vi "BonOMM-SAOMM.vi"() -> ()   [LabVIEW 2019] (continued)
                    n5983 = call "format_arcmin2arcsecstr.vi"("RA arcmin"=w2817, "DEC Arcmin"=w2816) -> ("Formatted RA"=w2820:string, "Formatted Dist"=w2818:string, "Formatted DEC"=w2819:string)  [unwired: 11 in]
                    n5984 = Array Max & Min(array=w2824) -> (max value=w2825:sgl)  [unwired: 3 out]
                    n5985 = call "Draw_crosshair.vi"("Image IN"=w2824, "White Value"=w2825) -> ("Image OUT"=w2823:sgl[][])  [unwired: 13 in]
                    n5986 = local write "SubIMG4DSS?"(TRUE ("SubIMG4DSS?")) -> ()
                    n5987 = local write "Cen-Cib-TOT"(w2818) -> ()
                    n5988 = local write "Cen-Cib-RA"(w2820) -> ()
                    n5989 = local write "Cen-Cib-DEC"(w2819) -> ()
                    n5990 = local write "ImageUsage"(w2808) -> ()
                    n5991 = local write "subimg"(w2823) -> ()
                  }
                  frame 4 {
                    # "À confirmer ..."
                    # "On envoie toujours les coordonnées en JNOW puisque Starry Night\nn'est pas capable de précesser des coordonnées correctement."
                    # "Synchroniser les coordonnées du télescope"
                    n5992 = local write "NO epoch"(w2838) -> ()
                    n5993 = expression code="x/3600."(w2841) -> (w2849:dbl)
                    n5994 = local write "N.O. A.D."(w2837) -> ()
                    n5995 = local write "N.O. Déc."(w2836) -> ()
                    n5996 = expression code="x/3600."(w2842) -> (w2848:dbl)
                    n5997 = Build Array(w2848, w2849, w2838) -> (w2850:dbl[])
                    n5998 = control-ref of="TCS actif"() -> (w2843:refnum<vi>)
                    n5999 = local read "TCS VRN"() -> (w2844:refnum<visa-resource-name>)
                    n6000 = call "EXCOM-CMD.vi"("VRN IN"=w2844, "Bool Refnum"=w2843, "Commande #"=6, "Args"=w2850) -> ("VRN OUT"=w2847:refnum<visa-resource-name>, "Error OUT"=w2846:errorcluster)  [unwired: 9 in, 1 out]
                    n6001 = local write "TCS Error"(w2846) -> ()
                    n6002 = local write "TCS VRN"(w2847) -> ()
                    "NO HA" <- w2840
                    "NO AM" <- w2839
                  }
                }
              }
            }
            n6003 = Wait Until Next ms Multiple(millisecond multiple=u32 500) -> ()  [unwired: 1 out]
            n6004 = local read "Quit"() -> (w2739:bool)
          }
          "Synchro StarryNight" <- w980
        }
      }
      n6005 = local write "QuitInitialization"(TRUE ("QuitInitialization")) -> ()
    }
    frame #9 {
      # "Cloture"
      n6006 = global read "Globals.vi" "BonOMM VI Refnum"() -> (w7898:refnum<vi>)
      n6007 = stacked-sequence {
        tunnel: w7898 -> [w7904 _ _ w7962 _ _]
        tunnel: w7899 -> [_ w7931 _ _ _ _]
        frame #0 {
          w7905 = FALSE
          w7930 = bool[] [FALSE, FALSE, FALSE]  # Array Constant
          # "Gestion dans le menu à revoir ..."
          n6008 = property class="VI"(reference=w7904) -> ("Front Panel.PanelBounds"=→"Front Panel Window:Panel Bounds":T6, "Minimum Panel Size"=→"Front Panel Window:Minimum Size":T5)  [unwired: 1 in, 2 out]
          n6009 = property on="Pane" class="Pann"() -> ("Origin"=→"Origin":T5)  [unwired: 2 in, 2 out]
          n6010 = Current VI's Menubar() -> (w7912:refnum<k9>)
          n6011 = Get Menu Item Info(7:"Affichage" ("item tag"), 11:w7912) -> (5:w7911:string[])  [unwired: 1 in, 6 out]
          n6012 = local write "Status lamp"(w7930) -> ()
          n6013 = Index Array(array=w7911, index #1=0 ("indice"), index #2=1 ("indice"), index #3=2 ("indice"), index #4=3 ("indice"), index #5=4 ("indice"), index #6=7 ("indice")) -> (element #1=w7923:string, element #2=w7922:string, element #3=w7921:string, element #4=w7920:string, element #5=w7919:string, element #6=w7907:string)
          n6014 = local read "Calib VRN"() -> (w7929:refnum<visa-resource-name>)
          n6015 = Current VI's Menubar() -> (w7908:refnum<k9>)
          n6016 = call "Controle_des_lampe.vi"("VISA resource name"=w7929, "Status In"=w7930) -> ()  [unwired: 3 out]
          n6017 = Get Menu Item Info(7:w7923, 11:w7908) -> (4:w7928:bool)  [unwired: 1 in, 6 out]
          n6018 = Get Menu Item Info(7:w7922, 11:w7908) -> (4:w7927:bool)  [unwired: 1 in, 6 out]
          n6019 = Get Menu Item Info(7:w7921, 11:w7908) -> (4:w7926:bool)  [unwired: 1 in, 6 out]
          n6020 = Get Menu Item Info(7:w7920, 11:w7908) -> (4:w7925:bool)  [unwired: 1 in, 6 out]
          n6021 = Get Menu Item Info(7:w7919, 11:w7908) -> (4:w7924:bool)  [unwired: 1 in, 6 out]
          n6022 = Get Menu Item Info(7:w7907, 11:w7908) -> (4:w7906:bool)  [unwired: 1 in, 6 out]
          n6023 = Build Array(w7928, w7927, w7926, w7925, w7924, w7905, w7905, w7906) -> (→"Éléments cochés":bool[])
        }
        frame #1 {
          n6024 = case shown="Vrai" w7931 {
            frame False {
            }
            frame True {
              n6025 = local read "Table VRN"() -> (w7941:refnum<visa-resource-name>)
              n6026 = VISA Close(VISA resource name=w7941) -> (error out=w7936:errorcluster)  [unwired: 1 in]
              n6027 = local write "Table Error"(w7936) -> ()
              n6028 = global read "Globals.vi" "CameraTuning VI Refnum"() -> (w7939:refnum<vi>)
              n6029 = local read "TCS VRN"() -> (w7945:refnum<visa-resource-name>)
              n6030 = global read "Globals.vi" "ScopeSim._Telescope"() -> (w7940:refnum<k7>)
              n6031 = VISA Close(VISA resource name=w7945) -> (error out=w7935:errorcluster)  [unwired: 1 in]
              n6032 = local read "PrAMS VRN"() -> (w7944:refnum<visa-resource-name>)
              n6033 = Close Reference(reference=w7940) -> (error out=w7937:errorcluster)  [unwired: 1 in]
              n6034 = Close Reference(reference=w7939) -> (error out=w7938:errorcluster)  [unwired: 1 in]
              n6035 = local write "Starry Night Error"(w7937) -> ()
              n6036 = local write "VI Reference Error"(w7938) -> ()
              n6037 = VISA Close(VISA resource name=w7944, error in (no error)=w7935) -> (error out=w7934:errorcluster)
              n6038 = local read "Excmd VRN"() -> (w7943:refnum<visa-resource-name>)
              n6039 = local write "TCS Error"(w7934) -> ()
              n6040 = VISA Close(VISA resource name=w7943) -> (error out=w7933:errorcluster)  [unwired: 1 in]
              n6041 = local read "Calib VRN"() -> (w7942:refnum<visa-resource-name>)
              n6042 = local write "Excom Error"(w7933) -> ()
              n6043 = VISA Close(VISA resource name=w7942) -> (error out=w7932:errorcluster)  [unwired: 1 in]
              n6044 = local write "Serial Error"(w7932) -> ()
            }
          }
        }
        frame #2 {
          # "Remplacer par un VI qui gère la déconnexion de PrAMS et Hexapode-Console"
          n6045 = disable-structure shown="Disabled" {
            frame Disabled {
              n6046 = local read "MessageType"() -> (w7948:cluster{string[], u32[]})
              n6047 = control-ref of="PrAMS-ACK"() -> (w7951:refnum<vi>)
              n6048 = control-ref of="PrAMS actif"() -> (w7952:refnum<vi>)
              n6049 = local read "PrAMS Error"() -> (w7949:errorcluster)
              n6050 = local read "PrAMS VRN"() -> (w7953:refnum<visa-resource-name>)
              n6051 = local read "Signature"() -> (w7950:u32)
              n6052 = call "SAOMM-SendSET.vi"("PRAMMS-COMM IN"=w7953, "Active Refnum"=w7952, "PrAMS-ACK"=w7951, "Signature"=w7950, "Error IN"=w7949, "MessageType"=w7948, "Active SET"="emtStopAcquisition", "Value (little endianed byte array)"=u8[] []) -> ()  [unwired: 4 in, 4 out]
            }
            frame Enabled {
            }
          }
        }
        frame #3 {
          # "Enregistrement de l'état des contrôles et indicateurs\ndans les fichiers controls.data et indicators.data"
          n6053 = local read "path_config"() -> (w7955:path)
          n6054 = invoke class="VI" method="ValCmde.TtObt"(reference=w7962, "Controls"=TRUE ("controls")) -> (reference out=w7979:refnum<vi>, error out=w7973:errorcluster, "Get All Control Values Variant"=w7961:cluster{"Name":string, "Variant Data":variant}[])  [unwired: 2 in, 1 out]
          n6055 = Build Path(base path=w7955, name or relative path="controls.data") -> (appended path=w7968:path)
          n6056 = Delete(path (use dialog)=w7968) -> (deleted path=w7967:path)  [unwired: 4 in, 2 out]
          n6057 = Flatten To String(anything=w7961) -> (data string=w7972:string)  [unwired: 3 in, 2 out]
          n6058 = for {
            tunnel: w7961 -> [w7981] mode=indexing
            tunnel: [w7980] -> w7960 mode=indexing
            n6059 = Unbundle(w7981) -> ("Name"=w7980:string)  [unwired: 1 out]
          }
          n6060 = call "Write Characters To File (no popup).vi"("append to file? (new file:F)"=FALSE, "character string"=w7972, "file path (dialog if empty)"=w7967) -> ()  [unwired: 2 in, 1 out]
          n6061 = local read "CtrlName"() -> (w7959:string[])
          n6062 = Not Equal?(x=w7959, y=w7960) -> (x != y?=w7958:bool[])
          n6063 = Boolean Array To Number(Boolean array=w7958) -> (number=w7957:u32)
          n6064 = invoke class="VI" method="ValCmde.TtObt"(reference=w7979, error in=w7973, "Controls"=FALSE ("controls")) -> (reference out=w7964:refnum<vi>, error out=w7963:errorcluster, "Get All Control Values Variant"=w7974:cluster{"Name":string, "Variant Data":variant}[])  [unwired: 1 in, 1 out]
          n6065 = Greater Than 0?(x=w7957) -> (x > 0?=w7956:bool)
          n6066 = local write "CtrlGetErrInd"(w7956) -> ()
          n6067 = Build Path(base path=w7955, name or relative path="indicators.data") -> (appended path=w7966:path)
          n6068 = Delete(path (use dialog)=w7966) -> (deleted path=w7965:path)  [unwired: 4 in, 2 out]
          n6069 = Flatten To String(anything=w7974) -> (data string=w7971:string)  [unwired: 3 in, 2 out]
          n6070 = call "Write Characters To File (no popup).vi"("append to file? (new file:F)"=FALSE, "character string"=w7971, "file path (dialog if empty)"=w7965) -> ()  [unwired: 2 in, 1 out]
          n6071 = Close Reference(reference=w7964, error in (no error)=w7963) -> (error out=w7954:errorcluster)
          n6072 = local write "Config Error"(w7954) -> ()
        }
        frame #4 {
          w7991 = "LVDTs" ("key")
          w7999 = i16 3 ("precision (6)")
          w8000 = T64."exponential" ("format (fractional)")
          w8006 = "tables"
          w8001 = "variables"
          # "Enregistrement dans le fichier \"properties.ini\""
          n6073 = local read "properties.ini"() -> (w8023:path)
          n6074 = call <vilib>:"Open Config Data.vi"("create file if necessary (T)"=FALSE, "configuration file path"=w8023) -> ("error out"=w8024:errorcluster, "refnum"=w8025:T23)  [unwired: 7 in, 1 out]
          n6075 = local read "k0_focus"() -> (w8057:dbl)
          n6076 = call-poly <vilib>:"Write Key.vi"("section"=w8001, "error in (no error)"=w8024, "value"=w8057, "key"="k0_focus", "refnum"=w8025) -> ("error out"=w8051:errorcluster, "refnum out"=w8055:T23)  [unwired: 4 in, 1 out]
          n6077 = local read "k1_focus"() -> (w8047:dbl)
          n6078 = call-poly <vilib>:"Write Key.vi"("section"=w8001, "error in (no error)"=w8051, "value"=w8047, "key"="k1_focus", "refnum"=w8055) -> ("error out"=w8050:errorcluster, "refnum out"=w8054:T23)  [unwired: 4 in, 1 out]
          n6079 = local read "a1_focus"() -> (w8045:dbl)
          n6080 = call-poly <vilib>:"Write Key.vi"("format (fractional)"=w8000, "precision (6)"=w7999, "section"=w8001, "error in (no error)"=w8050, "value"=w8045, "key"="a1_focus", "refnum"=w8054) -> ("error out"=w8049:errorcluster, "refnum out"=w8053:T23)  [unwired: 2 in, 1 out]
          n6081 = local read "a2_focus"() -> (w8042:dbl)
          n6082 = call-poly <vilib>:"Write Key.vi"("format (fractional)"=w8000, "precision (6)"=w7999, "section"=w8001, "error in (no error)"=w8049, "value"=w8042, "key"="a2_focus", "refnum"=w8053) -> ("error out"=w8048:errorcluster, "refnum out"=w8052:T23)  [unwired: 2 in, 1 out]
          n6083 = local read "a3_focus"() -> (w8040:dbl)
          n6084 = call-poly <vilib>:"Write Key.vi"("format (fractional)"=w8000, "precision (6)"=w7999, "section"=w8001, "error in (no error)"=w8048, "value"=w8040, "key"="a3_focus", "refnum"=w8052) -> ("error out"=w7982:errorcluster, "refnum out"=w7983:T23)  [unwired: 2 in, 1 out]
          n6085 = local read "dflt-EQX"() -> (w8002:dbl)
          n6086 = call-poly <vilib>:"Write Key.vi"("section"=w8001, "error in (no error)"=w7982, "value"=w8002, "key"="equinox", "refnum"=w7983) -> ("error out"=w7994:errorcluster, "refnum out"=w7998:T23)  [unwired: 4 in, 1 out]
          n6087 = local read "LVDT-zero"() -> (w7984:dbl)
          n6088 = call-poly <vilib>:"Write Key.vi"("section"=w7991, "error in (no error)"=w7994, "value"=w7984, "key"="ra-zero", "refnum"=w7998) -> ("error out"=w7993:errorcluster, "refnum out"=w7997:T23)  [unwired: 4 in, 1 out]
          n6089 = local read "LVDT-scale"() -> (w7986:dbl)
          n6090 = call-poly <vilib>:"Write Key.vi"("section"=w7991, "error in (no error)"=w7993, "value"=w7986, "key"="ra-scale", "refnum"=w7997) -> ("error out"=w7992:errorcluster, "refnum out"=w7996:T23)  [unwired: 4 in, 1 out]
          n6091 = local read "LVDT-time"() -> (w7985:dbl)
          n6092 = call-poly <vilib>:"Write Key.vi"("section"=w7991, "error in (no error)"=w7992, "value"=w7985, "key"="acq-time", "refnum"=w7996) -> ("error out"=w7987:errorcluster, "refnum out"=w7995:T23)  [unwired: 4 in, 1 out]
          n6093 = local read "vitesse rapide"() -> (w8017:dbl)
          n6094 = call-poly <vilib>:"Write Key.vi"("section"=w8006, "error in (no error)"=w7987, "value"=w8017, "key"="vrapid", "refnum"=w7995) -> ("error out"=w8010:errorcluster, "refnum out"=w8012:T23)  [unwired: 4 in, 1 out]
          n6095 = local read "vitesse lente"() -> (w8018:dbl)
          n6096 = call-poly <vilib>:"Write Key.vi"("section"=w8006, "error in (no error)"=w8010, "value"=w8018, "key"="vlente", "refnum"=w8012) -> ("error out"=w8009:errorcluster, "refnum out"=w8011:T23)  [unwired: 4 in, 1 out]
          n6097 = local read "accelleration"() -> (w8019:dbl)
          n6098 = call-poly <vilib>:"Write Key.vi"("section"=w8006, "error in (no error)"=w8009, "value"=w8019, "key"="accel", "refnum"=w8011) -> ("error out"=w8020:errorcluster, "refnum out"=w8021:T23)  [unwired: 4 in, 1 out]
          n6099 = local read "vitesse focus"() -> (w8022:dbl)
          n6100 = call-poly <vilib>:"Write Key.vi"("section"=w8006, "error in (no error)"=w8020, "value"=w8022, "key"="vfocus", "refnum"=w8021) -> ("error out"=w8007:errorcluster, "refnum out"=w8008:T23)  [unwired: 4 in, 1 out]
          n6101 = local read "CentreTel X"() -> (w8031:dbl)
          n6102 = call-poly <vilib>:"Write Key.vi"("section"=w8006, "error in (no error)"=w8007, "value"=w8031, "key"="cenx", "refnum"=w8008) -> ("error out"=w8038:errorcluster, "refnum out"=w8036:T23)  [unwired: 4 in, 1 out]
          n6103 = local read "CentreTel Y"() -> (w8030:dbl)
          n6104 = call-poly <vilib>:"Write Key.vi"("section"=w8006, "error in (no error)"=w8038, "value"=w8030, "key"="ceny", "refnum"=w8036) -> ("error out"=w8039:errorcluster, "refnum out"=w8037:T23)  [unwired: 4 in, 1 out]
          n6105 = local read "Reference X"() -> (w8029:dbl)
          n6106 = call-poly <vilib>:"Write Key.vi"("section"=w8006, "error in (no error)"=w8039, "value"=w8029, "key"="refX", "refnum"=w8037) -> ("error out"=w8028:errorcluster, "refnum out"=w8027:T23)  [unwired: 4 in, 1 out]
          n6107 = local read "Reference Y"() -> (w8026:dbl)
          n6108 = call-poly <vilib>:"Write Key.vi"("section"=w8006, "error in (no error)"=w8028, "value"=w8026, "key"="refY", "refnum"=w8027) -> ("error out"=w8004:errorcluster, "refnum out"=w8005:T23)  [unwired: 4 in, 1 out]
          n6109 = call <vilib>:"Close Config Data.vi"("error in (no error)"=w8004, "refnum"=w8005) -> ()  [unwired: 8 in, 2 out]
        }
        frame #5 {
          n6110 = call "Enregistrement des parametres.vi"() -> ()  [unwired: 1 in]
        }
      }
      n6111 = case shown="Vrai" w7897 {
        selector: w7897 -> [_ w7900]
        frame False {
        }
        frame True {
          n6112 = property on="filtre_nom" class="Ch"("Visible"=w7900) -> ()  [unwired: 2 in, 2 out]
          n6113 = property on="q-raf" class="Bool (strict)"("Visible"=w7900) -> ()  [unwired: 2 in, 2 out]
          n6114 = property on="cancel-raf" class="Bool (strict)"("Visible"=w7900) -> ()  [unwired: 2 in, 2 out]
          n6115 = property on="change_filtre_liste" class="Bool (strict)"("Visible"=w7900) -> ()  [unwired: 2 in, 2 out]
          n6116 = property on="StopCam" class="Bool (strict)"("Visible"=w7900) -> ()  [unwired: 2 in, 2 out]
          n6117 = property on="GoCam" class="Bool (strict)"("Visible"=w7900) -> ()  [unwired: 2 in, 2 out]
          n6118 = property on="F#" class="NumNb (strict)"("Visible"=w7900) -> ()  [unwired: 2 in, 2 out]
          n6119 = property on="ChoixFiltre" class="Clust (strict)"("Visible"=w7900) -> ()  [unwired: 2 in, 2 out]
          n6120 = property on="ST_RAZ" class="Bool"("Visible"=w7900) -> ()  [unwired: 2 in, 2 out]
          n6121 = property on="ST-" class="Bool (strict)"("Visible"=w7900) -> ()  [unwired: 2 in, 2 out]
          n6122 = property on="ST+" class="Bool (strict)"("Visible"=w7900) -> ()  [unwired: 2 in, 2 out]
          n6123 = property on="SET ZERO" class="Bool"("Visible"=w7900) -> ()  [unwired: 2 in, 2 out]
        }
      }
      n6124 = property on="Approaching limit" class="Bool (strict)"("Visible"=w7897, "Blinking"=w7897) -> ()  [unwired: 2 in, 2 out]
      n6125 = property on="Target OutofRange" class="Bool (strict)"("Visible"=w7897, "Blinking"=w7897) -> ()  [unwired: 2 in, 2 out]
    }
  }
